vi "Calc_angles_and_ratios.vi"(7 "COS ratio (TO/FROM) - internal":dbl=0.99999, 10 "Refr index":dbl=7.5, 11 "Angle FROM deg (ext)":dbl=7.5) -> (0 "V at angle TO":dbl=209.7885634804175, 1 "V at angle FROM":dbl=209.7885634804175, 2 "Cos  FROM  (internal)":dbl=0.9993007047883986, 3 "Angle TO  deg (ext)":dbl=6.959125577482326)   [LabVIEW 2010]
panel:
  out "CosTO (internal)":dbl=0.9993007047883986
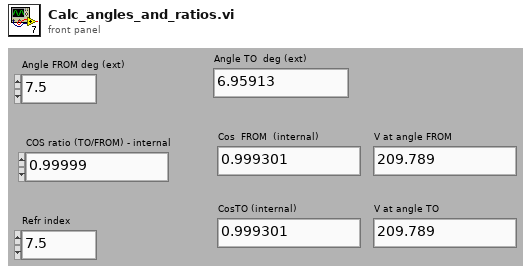
[diagram p1: front panel]
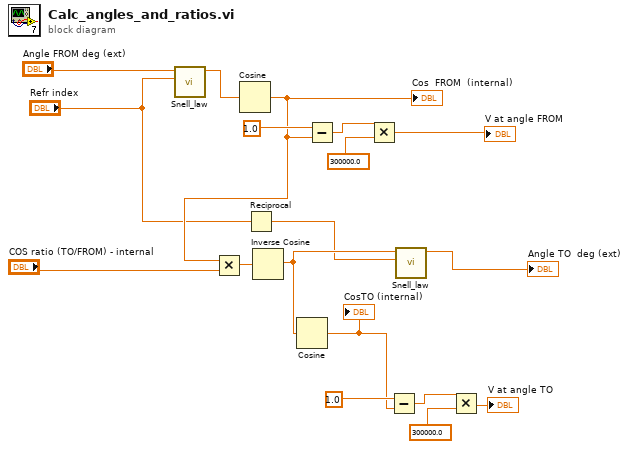
[diagram p0: block diagram]
diagram:
  n1 = call "Snell_law.vi"("Refr index"="Refr index", "Angle in ext (deg)"="Angle FROM deg (ext)") -> ("Angle out int (rad)"=w5:dbl)  [unwired: 8 in, 1 out]
  n2 = Cosine(x=w5) -> (cos(x)=w15:dbl)
  "Cos  FROM  (internal)" <- w15
  n3 = Multiply(x=w15, y="COS ratio (TO/FROM) - internal") -> (x*y=w9:dbl)
  n4 = Reciprocal(x="Refr index") -> (1/x=w2:dbl)
  n5 = Inverse Cosine(1:w9) -> (0:w4:dbl)
  n6 = Cosine(x=w4) -> (cos(x)=w7:dbl)
  "CosTO (internal)" <- w7
  n7 = Subtract(x=sgl 1.0, y=w15) -> (x-y=w16:dbl)
  n8 = Multiply(x=w16, y=sgl 300000.0) -> (x*y=→"V at angle FROM":dbl)
  n9 = Subtract(x=sgl 1.0, y=w7) -> (x-y=w13:dbl)
  n10 = call "Snell_law.vi"("Refr index"=w2, "Angle in ext (deg)"=w4) -> ("Angle out int (rad)"=→"Angle TO  deg (ext)":dbl)  [unwired: 8 in, 1 out]
  n11 = Multiply(x=w13, y=sgl 300000.0) -> (x*y=→"V at angle TO":dbl)
